vi "SampleRelativeMove_8742.vi"() -> ()   [LabVIEW 2009]
panel:
  in  "Relative Steps":i32
  in  "Motor Number":i32=1
  in  "stop":bool
  out "Position Status":i32
  out "error out":errorcluster
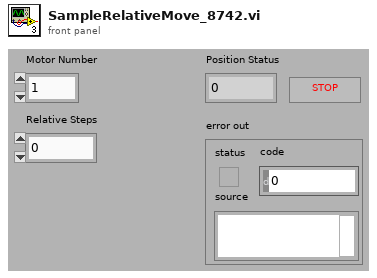
[diagram p1: front panel]
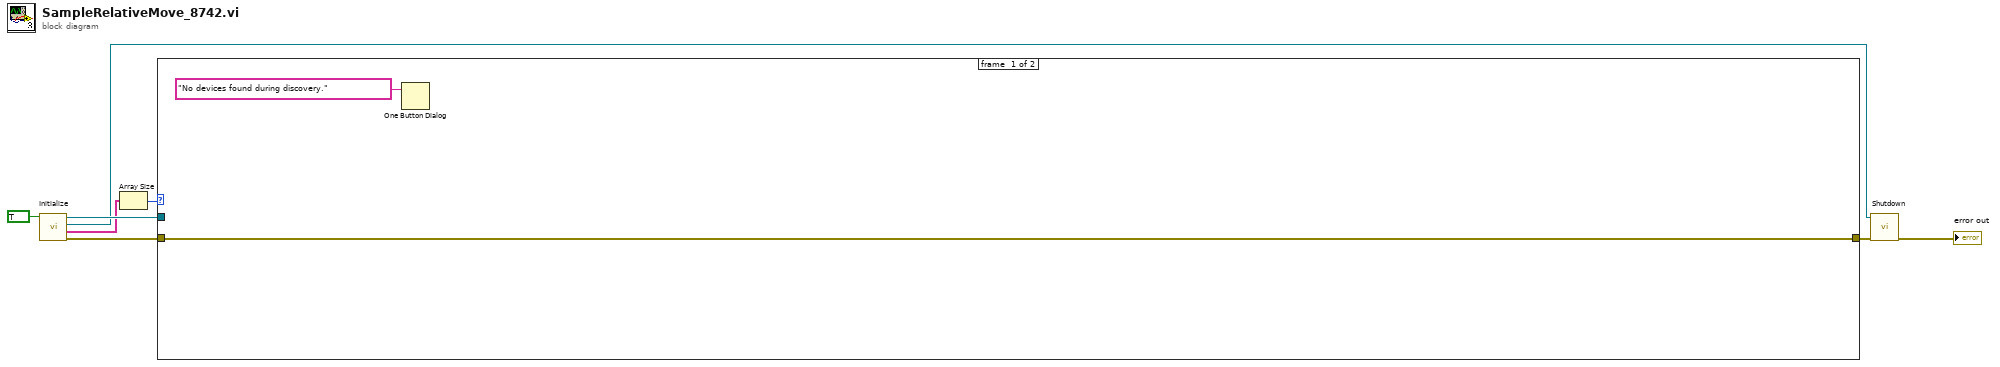
[diagram p0: block diagram]
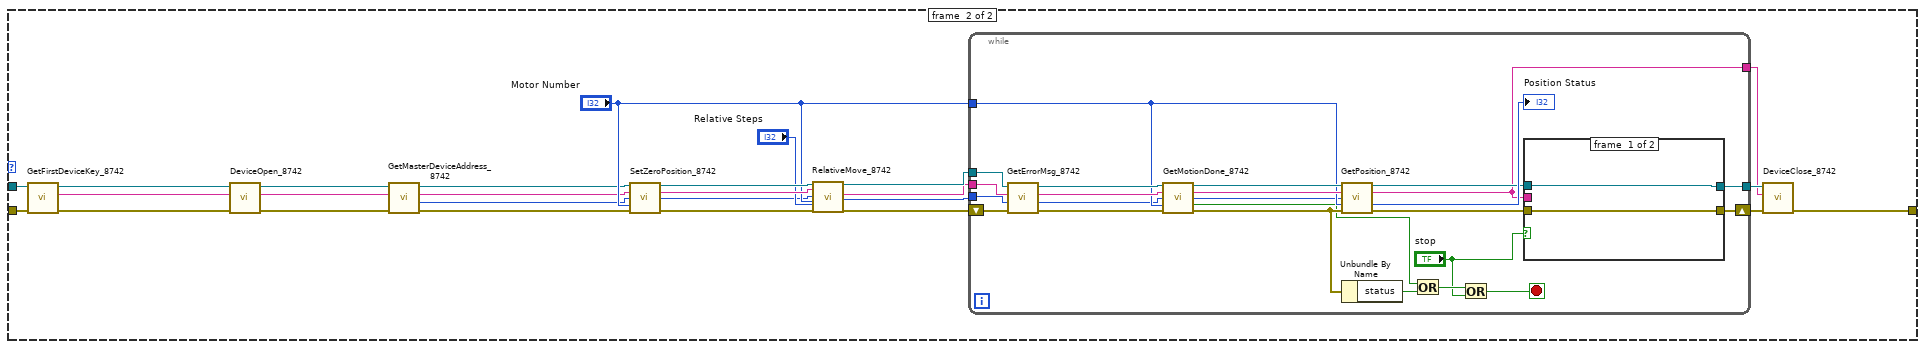
[diagram p2: hidden frame]
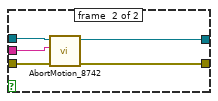
[diagram p3: hidden frame]
diagram:
  n1 = call "Initialize.vi"("logging"=TRUE) -> ("error out"=w3:errorcluster, "DeviceKey List"=w2:string[], "DeviceIOLib Out"=w1:refnum<k24>, "CmdLib Out"=w5:refnum<k24>)  [unwired: 3 in]
  n2 = Array Size(array=w2) -> (size(s)=w4:i32)
  n3 = case shown="1, Default" w4 {
    tunnel: [w9 w12] -> w6
    tunnel: w5 -> [_ w21]
    tunnel: w3 -> [w9 w22]
    frame #0 {
      n4 = One Button Dialog(message="No devices found during discovery.") -> ()  [unwired: 1 in, 1 out]
    }
    frame #1 {
      n5 = call "GetFirstDeviceKey_8742.vi"("error in"=w22, "CmdLib In"=w21) -> ("error out"=w20:errorcluster, "DeviceKey Out"=w18:string, "CmdLib Out"=w16:refnum<k24>)  [unwired: 3 in]
      n6 = call "DeviceOpen_8742.vi"("error in (no error)"=w20, "DeviceKey In"=w18, "CmdLib In"=w16) -> ("error out"=w19:errorcluster, "DeviceKey Out"=w17:string, "CmdLib Out"=w15:refnum<k24>)  [unwired: 2 in]
      n7 = call "GetMasterDeviceAddress_8742.vi"("error in (no error)"=w19, "DeviceKey In"=w17, "CmdLib In"=w15) -> ("error out"=w27:errorcluster, "Device Address"=w28:i32, "DeviceKey Out"=w25:string, "CmdLib Out"=w26:refnum<k24>)  [unwired: 1 in]
      n8 = call "SetZeroPosition_8742.vi"("CmdLib In"=w26, "DeviceKey In"=w25, "Device Address In"=w28, "Motor"="Motor Number", "error in (no error)"=w27) -> ("CmdLib Out"=w33:refnum<k24>, "DeviceKey Out"=w32:string, "Device Address Out"=w24:i32, "error out"=w31:errorcluster)  [unwired: 7 in]
      n9 = call "RelativeMove_8742.vi"("CmdLib In"=w33, "DeviceKey In"=w32, "Device Address In"=w24, "Motor"="Motor Number", "Relative Steps"="Relative Steps", "error in (no error)"=w31) -> ("CmdLib Out"=w36:refnum<k24>, "DeviceKey Out"=w35:string, "Device Address Out"=w23:i32, "error out"=w34:errorcluster)  [unwired: 10 in]
      n10 = while {
        tunnel: "Motor Number" -> [w56]
        tunnel: w36 -> [w55]
        tunnel: w35 -> [w54]
        tunnel: [w41] -> w14
        tunnel: w23 -> [w40]
        shift-right: [w43] -> w13
        shift-left: w34 -> [w53]
        tunnel: [w37] -> w11
        stop <- w46 stop-if-true
        n11 = call "GetErrorMsg_8742.vi"("error in (no error)"=w53, "Device Address In"=w40, "DeviceKey In"=w54, "CmdLib In"=w55) -> ("error out"=w52:errorcluster, "Device Address Out"=w39:i32, "DeviceKey Out"=w58:string, "CmdLib Out"=w57:refnum<k24>)
        n12 = call "GetMotionDone_8742.vi"("CmdLib In"=w57, "DeviceKey In"=w58, "Device Address In"=w39, "Motor"=w56, "error in (no error)"=w52) -> ("CmdLib Out"=w59:refnum<k24>, "DeviceKey Out"=w60:string, "Device Address Out"=w38:i32, "Is Motion Done"=w49:bool, "error out"=w50:errorcluster)  [unwired: 6 in]
        n13 = call "GetPosition_8742.vi"("CmdLib In"=w59, "DeviceKey In"=w60, "Device Address In"=w38, "Motor"=w56, "error in (no error)"=w50) -> ("CmdLib Out"=w42:refnum<k24>, "DeviceKey Out"=w37:string, "Position"=→"Position Status":i32, "error out"=w44:errorcluster)  [unwired: 6 in, 1 out]
        n14 = Unbundle By Name(w50) -> ("status"=w51:bool)
        n15 = Or(x=w49, y=w51) -> (x .or. y?=w47:bool)
        n16 = Or(x=w47, y="stop") -> (x .or. y?=w46:bool)
        n17 = case shown="True" "stop" {
          tunnel: w44 -> [w61 w67]
          tunnel: [w61 w66] -> w43
          tunnel: w42 -> [w62 w65]
          tunnel: [w62 w64] -> w41
          tunnel: w37 -> [_ w63]
          frame #0 {
          }
          frame #1 {
            n18 = call "AbortMotion_8742.vi"("error in (no error)"=w67, "DeviceKey In"=w63, "CmdLib In"=w65) -> ("error out"=w66:errorcluster, "CmdLib Out"=w64:refnum<k24>)  [unwired: 1 in, 2 out]
          }
        }
      }
      n19 = call "DeviceClose_8742.vi"("error in (no error)"=w13, "DeviceKey In"=w11, "CmdLib In"=w14) -> ("error out"=w12:errorcluster)  [unwired: 2 in, 2 out]
    }
  }
  n20 = call "Shutdown.vi"("error in (no error)"=w6, "DeviceIOLib In"=w1) -> ("error out"=→"error out":errorcluster)  [unwired: 5 in]
